vi "WS1050 16 DUT VSA-CV Sweep HD_Cycling_Ver1.0.vi"() -> ()   [LabVIEW 2012]
uses:
  Type Defs/WSVCAP SHL I2C DUT Mask Mode Enum.ctl
  <vilib>/Utility/file.llb/Read From Spreadsheet File (DBL).vi
  SubVI/Agilent E363X Series/Agilent E363X Series.lvlib
  SubVI/keithley_2000/Keithley 2000/Keithley 2000.lvlib
  SubVI/2012_Keithley 24XX/Keithley 24XX.lvlib
panel:
  out "VISA resource name out":refnum<visa-resource-name>="GPIB0::3::INSTR"
  out "date string":string="5/19/2014"
  out "PS1 Out":refnum<visa-resource-name>
  out "Ke2000 Out":refnum<visa-resource-name>="GPIB0::9::INSTR"
  in  "Tab Control":enum32{"Inst Control", "Data Output", "Graphs"}(tab)
  out "AD7747 Values":string[][](table)
  in  "Lot#":string="4NEMB"
  in  "Wafer#":string="20-EB"
  in  "File Name":string="HD_4NEMB_25_EB_65C_44V_100DC_BRD2_150916_1"
  in  "TMN DC\\CAP Data Log File Path":path=path "C:/WS1050 16 DUT Data"
  in  "SN":string[](array[string])=["1", "2", "3", "4", "5", "6", "7", "8", "9", "10", "11", "12", "13", "14", "15", "16"]
  in  "Test Program":string="WS1050 16 DUT VSA_CV Sweep HD_Cycling Ver1.0"
  out "Current Date":string="8/28/2014"
  out "Current Time":string="0950"
  in  "Start Date":string="4/24/2014"
  in  "Start Time":string="1542"
  in  "Comment":string="VSA CV Sweep"
  in  "OK Button":bool
  in  "Calibration":bool
  in  "Control Setting":bool
  in  "CP Setting":i32(ring) items=["CP OFF", "CP ON", "CP 35V", "CP 40V", "CP 44V", "CP 50V", "DVA OFF", "DVA ON", "Reg1 ON", "Reg1 OFF", "Reg2 ON", "Reg2 OFF", "Reg3 ON", "Reg3 OFF"]
  in  "VDD(V)":dbl=3.3 format="%.3g"
  in  "SPI Clock Rate (Hz)":dbl=1000000.0 caption="Meas Speed" format="%.1p Hz"
  out "AR  Measurent(Hz)":dbl
  in  "PS1 Source":refnum<visa-resource-name>="GPIB0::5::INSTR"
  in  "Ke2000":refnum<visa-resource-name>="GPIB0::9::INSTR"
  out "Simulate FPGA":bool
  out "Online":bool
  in  "Ke2400":refnum<visa-resource-name>="GPIB0::3::INSTR"
  in  "Initialize AD7747":bool
  in  "DUT Mask Mode":T1=enum."All"
  in  "RFFE Slave Address":u8=7 caption="Slave Address" format="0x%02x"
  out "Activity Log":string="05/19/2014 -- 12:24:35.853::WSVCAP::APP::Application Started\n05/19/2014 -- 12:24:37.606::WSVCAP::WSVCAP SHL::WR I2C-REG:0x0A;MASK:0xFFFFFFFFFFFF;C1 DATA:22:22:22:22:22:22:22:22:22:22:22:22:22:22:22:22;C2 DATA:22:22:22:22:22:22:22:22:22:22:22:22:22:22:22:22;C3 DATA:22:22:22:22:22:22:22:22:22:22:22:22:22:22:22:22\r\n05/19/2014 -- 12:24:37.773::WSVCAP::WSVCAP SHL::WR I2C-ST:0,0,4,1\r\n05/19/2014 -- 12:24:37.903::WSVCAP::WSVCAP SHL::RD I2C-BYTES:4;ADD:0x00;MASK:0xFFFFFFFFFFFF\r\n05/19/2014 -- 12:24:38.045::WSVCAP::WSVCAP SHL::RD I2C:C1 DATA:2:2:2:2:2:2:2:2:2:2:2:2:2:2:2:2|A7:A9:AA:82:82:7F:82:81:82:81:83:82:81:82:82:81|46:36:BB:88:44:A3:E9:2B:32:20:ED:25:BB:3D:68:B|2C:6A:EB:A7:22:56:FE:CC:36:82:D7:B0:3B:48:F9:CC;C2 DATA:2:2:2:2:2:2:2:2:2:2:2:2:2:2:2:2|94:94:94:80:80:80:80:80:81:7E:7E:81:80:7E:80:80|47:33:15:82:62:B:E8:1C:D7:C3:7D:41:7C:B7:4C:2A|C4:B4:AE:8:1E:D1:4E:37:11:C0:6F:63:42:9D:63:B5;C3 DATA:2:2:2:2:2:2:2:2:2:2:2:2:2:2:2:2|95:95:95:81:81:7E:81:80:84:7D:80:83:81:7E:7F:80|AB:C4:14:B5:7B:52:DF:C9:79:5D:5F:30:99:31:1E:F4|6E:5C:F7:A8:C3:EB:7B:EF:33:92:89:77:4D:67:75:DD;STATUS:0:0:4:0\r\n05/19/2014 -- 12:24:38.046::WSVCAP::WSVCAP SHL::WR I2C-REG:0x0A;MASK:0xFFFFFFFFFFFF;C1 DATA:22:22:22:22:22:22:22:22:22:22:22:22:22:22:22:22;C2 DATA:22:22:22:22:22:22:22:22:22:22:22:22:22:22:22:22;C3 DATA:22:22:22:22:22:22:22:22:22:22:22:22:22:22:22:22\r\n05/19/2014 -- 12:24:38.089::WSVCAP::WSVCAP SHL::WR I2C-ST:0,0,4,1\r\n05/19/2014 -- 12:24:38.219::WSVCAP::WSVCAP SHL::RD I2C-BYTES:4;ADD:0x00;MASK:0xFFFFFFFFFFFF\r\n05/19/2014 -- 12:24:38.362::WSVCAP::WSVCAP SHL::RD I2C:C1 DATA:2:2:2:2:2:2:2:2:2:2:2:2:2:2:2:2|A7:AB:AA:82:82:82:83:83:82:82:82:82:7F:82:82:81|4B:32:96:83:3E:61:43:17:25:62:AB:4D:A2:40:2E:5|3C:76:2B:B4:EE:E4:A9:1A:AA:A:26:C7:21:2E:87:5B;C2 DATA:2:2:2:2:2:2:2:2:2:2:2:2:2:2:2:2|94:94:94:80:80:80:80:80:80:7F:80:81:80:80:7F:80|4A:32:19:7D:19:6C:79:46:61:7F:4B:B8:A5:30:F3:14|B4:70:A:8C:9C:DC:43:FA:1E:A:C6:21:A:A9:13:F3;C3 DATA:2:2:2:2:2:2:2:2:2:2:2:2:2:2:2:2|95:97:94:81:80:81:82:81:80:7E:81:84:7F:81:80:80|B2:32:D0:A7:9E:4C:AB:D4:EE:D9:F0:82:B7:91:7:FF|C1:91:B6:3D:D8:E:1B:4F:9F:6A:F1:6C:E7:3F:7:BA;STATUS:0:0:4:0\r\n05/19/2014 -- 12:24:38.364::WSVCAP::WSVCAP SHL::WR I2C-REG:0x0A;MASK:0xFFFFFFFFFFFF;C1 DATA:22:22:22:22:22:22:22:22:22:22:22:22:22:22:22:22;C2 DATA:22:22:22:22:22:22:22:22:22:22:22:22:22:22:22:22;C3 DATA:22:22:22:22:22:22:22:22:22:22:22:22:22:22:22:22\r\n05/19/2014 -- 12:24:38.406::WSVCAP::WSVCAP SHL::WR I2C-ST:0,0,4,1\r\n05/19/2014 -- 12:24:38.536::WSVCAP::WSVCAP SHL::RD I2C-BYTES:4;ADD:0x00;MASK:0xFFFFFFFFFFFF\r\n05/19/2014 -- 12:24:38.678::WSVCAP::WSVCAP SHL::RD I2C:C1 DATA:2:2:2:2:2:2:2:2:2:2:2:2:2:2:2:2|A7:A9:AB:82:82:81:82:82:82:82:82:82:82:82:82:81|46:71:4C:87:43:3D:7F:FC:25:4F:8E:54:97:3E:60:8C|AA:F4:1F:B5:CE:43:1F:36:9:87:9C:78:86:5:B6:8E;C2 DATA:2:2:2:2:2:2:2:2:2:2:2:2:2:2:2:2|94:94:94:80:7F:7F:80:80:80:80:80:81:80:80:80:80|49:36:18:7D:6E:C5:E4:3C:81:2E:41:D3:75:71:E3:72|E8:D3:E6:D1:E0:48:AE:D4:54:D:E8:8E:B4:41:68:4;C3 DATA:2:2:2:2:2:2:2:2:2:2:2:2:2:2:2:2|95:95:95:81:7F:7F:81:81:81:81:81:84:81:81:82:81|B3:F5:90:AB:82:69:7B:93:D0:77:E8:D5:E8:8C:84:E8|B9:AC:EE:2B:B6:71:8F:4A:74:31:56:BB:8A:B7:A0:C8;STATUS:0:0:4:0\r\n05/19/2014 -- 12:24:38.681::WSVCAP::WSVCAP SHL::WR I2C-REG:0x0A;MASK:0xFFFFFFFFFFFF;C1 DATA:22:22:22:22:22:22:22:22:22:22:22:22:22:22:22:22;C2 DATA:22:22:22:22:22:22:22:22:22:22:22:22:22:22:22:22;C3 DATA:22:22:22:22:22:22:22:22:22:22:22:22:22:22:22:22\r\n05/19/2014 -- 12:24:38.723::WSVCAP::WSVCAP SHL::WR I2C-ST:0,0,4,1\r\n05/19/2014 -- 12:24:38.854::WSVCAP::WSVCAP SHL::RD I2C-BYTES:4;ADD:0x00;MASK:0xFFFFFFFFFFFF\r\n05/19/2014 -- 12:24:38.996::WSVCAP::WSVCAP SHL::RD I2C:C1 DATA:2:2:2:2:2:2:2:2:2:2:2:2:2:2:2:2|A7:A9:AA:82:82:7F:83:81:82:81:84:82:7F:82:7F:82|43:FB:E:7F:3C:AD:35:35:26:A2:6C:21:4B:3D:8:6|63:9A:E1:F3:95:32:91:42:90:3C:78:1F:5C:D7:5F:D8;C2 DATA:2:2:2:2:2:2:2:2:2:2:2:2:2:2:2:2|94:94:94:80:80:80:80:80:81:80:7E:81:80:7E:7F:80|48:36:18:7F:5E:3D:69:83:DE:AE:A1:9E:31:AE:BB:96|15:A0:44:17:13:FD:CC:C8:6D:B2:EF:A7:C:C7:3B:F;C3 DATA:2:2:2:2:2:2:2:2:2:2:2:2:2:2:2:2|95:96:94:81:81:7E:82:80:84:80:80:84:7F:7E:7D:82|AD:3B:6D:A9:7C:57:9D:F5:7A:96:23:5C:36:2D:ED:5A|CD:46:DB:3B:C7:BD:70:60:33:B8:B:F7:63:A:51:4D;STATUS:0:0:4:0\r\n05/19/2014 -- 12:24:38.998::WSVCAP::WSVCAP SHL::WR I2C-REG:0x0A;MASK:0xFFFFFFFFFFFF;C1 DATA:22:22:22:22:22:22:22:22:22:22:22:22:22:22:22:22;C2 DATA:22:22:22:22:22:22:22:22:22:22:22:22:22:22:22:22;C3 DATA:22:22:22:22:22:22:22:22:22:22:22:22:22:22:22:22\r\n05/19/2014 -- 12:24:39.040::WSVCAP::WSVCAP SHL::WR I2C-ST:0,0,4,1\r\n05/19/2014 -- 12:24:39.170::WSVCAP::WSVCAP SHL::RD I2C-BYTES:4;ADD:0x00;MASK:0xFFFFFFFFFFFF\r\n05/19/2014 -- 12:24:39.311::WSVCAP::WSVCAP SHL::RD I2C:C1 DATA:2:2:2:2:2:2:2:2:2:2:2:2:2:2:2:2|A7:AA:AB:82:82:81:82:81:82:81:82:82:82:82:7F:82|44:F1:90:87:45:44:C8:2C:2C:F1:FC:1B:94:3B:3C:75|4A:49:95:19:99:73:64:3:23:24:F3:A2:5E:7F:C4:B6;C2 DATA:2:2:2:2:2:2:2:2:2:2:2:2:2:2:2:2|94:94:94:80:80:80:80:7F:80:80:7E:80:80:7E:7F:80|4C:36:17:7D:A8:9F:DE:C7:53:6D:8A:F4:41:A5:C6:E0|90:2E:24:C:D9:22:E4:76:3B:40:1D:53:33:B1:3E:4D;C3 DATA:2:2:2:2:2:2:2:2:2:2:2:2:2:2:2:2|95:97:95:81:81:7F:81:80:80:81:7F:82:81:7E:7D:82|AE:2B:A7:AB:CC:CD:A4:38:FD:17:80:F2:92:2D:45:C4|76:E5:D:B9:AD:B5:BA:8D:28:32:9E:42:B7:20:4A:D9;STATUS:0:0:4:0\r\n05/19/2014 -- 12:24:39.313::WSVCAP::WSVCAP SHL::WR I2C-REG:0x0A;MASK:0xFFFFFFFFFFFF;C1 DATA:22:22:22:22:22:22:22:22:22:22:22:22:22:22:22:22;C2 DATA:22:22:22:22:22:22:22:22:22:22:22:22:22:22:22:22;C3 DATA:22:22:22:22:22:22:22:22:22:22:22:22:22:22:22:22\r\n05/19/2014 -- 12:24:39.355::WSVCAP::WSVCAP SHL::WR I2C-ST:0,0,4,1\r\n05/19/2014 -- 12:24:39.486::WSVCAP::WSVCAP SHL::RD I2C-BYTES:4;ADD:0x00;MASK:0xFFFFFFFFFFFF\r\n05/19/2014 -- 12:24:39.628::WSVCAP::WSVCAP SHL::RD I2C:C1 DATA:2:2:2:2:2:2:2:2:2:2:2:2:2:2:2:2|A7:A9:AA:82:82:82:83:82:82:82:82:82:7F:82:7F:82|47:18:E4:87:3E:E7:6:65:25:92:37:38:A8:3E:89:85|7C:A7:7:2B:A3:7A:EC:EF:89:ED:F4:D3:D8:BC:3A:F5;C2 DATA:2:2:2:2:2:2:2:2:2:2:2:2:2:2:2:2|94:94:94:80:7F:80:80:7F:81:80:7E:80:80:80:81:80|49:37:17:80:76:25:6A:F8:DF:55:97:4D:B8:5B:2B:B1|13:E3:9A:3E:1A:2D:4F:B6:DB:E9:61:FA:8B:D6:9:CC;C3 DATA:2:2:2:2:2:2:2:2:2:2:2:2:2:2:2:2|95:95:95:81:7F:80:82:81:84:80:7F:81:80:81:7F:82|AF:93:3B:AF:5B:11:82:E4:7E:C3:2D:72:9:96:D9:A|DB:96:F2:10:5F:64:9A:C6:98:12:27:7D:10:D3:20:D9;STATUS:0:0:4:0\r\n05/19/2014 -- 12:24:40.132::WSVCAP::WSVCAP SHL::CLOSE\r\n"
  in  "C1 Cap DAC":u8=128 caption="B Data In" format="0x%02x"
  in  "C2 Cap DAC":u8=128 caption="B Data In" format="0x%02x"
  in  "C3 Cap DAC":u8=128 caption="B Data In" format="0x%02x"
  out "IDD Brd(uA)":string
  in  "VSA_IDD(A)":dbl=0.1
  in  "Cmd to HD_ON":string="0702013B3B3B"
  in  "Stress Voltage(V)":dbl=10.0
  in  "error in (no error)":errorcluster
  out "error out":errorcluster
  in  "CP to HD/Cycle":i32(ring)=4 items=["CP HDC 35V", "CP HDC 40.25V", "CP HDC 27.5V", "CP HDC 30.5V", "CP HDC 44V", "CP HDC 50V"]
  out "STATUS":string="Idle...."
  in  "stop":bool
  out "VSA_C1_T0":string[](array[string])
  out "VSA_Value(pF)":string[][](array[string])
  out "VSA_C3_T0":string[](array[string])
  out "VSA_C2_T0":string[](array[string])
  in  "Abort":bool
  out "error out 2":errorcluster
  in  "Set HD Time \nto Complete(Min)":u64=259200
  out "HD Time\nCompleted(Min)":u64
  out "Verify Test Condition":string[](array[string])
  out "All CMin Current":string[][](table)
  out "Previous Time":string="12:20:26 PM"
  out "Running Loops":i32=1
  out "Verify Drivers to Stress":string[](array[string])
  out "VSA Delta C1(pF)":dbl[](array[numeric])
  out "VSA Delta C2(pF)":dbl[](array[numeric])
  out "VSA Delta C3(pF)":dbl[](array[numeric])
  out "CP Current(uA)":string[](array[string])
  out "Plot VSA Delta C3":cluster{dbl[], "VSA Delta C(pF)":dbl[]}(graph)
  out "Plot VSA Delta C2":cluster{dbl[], "VSA Delta C(pF)":dbl[]}(graph)
  out "Plot VSA Delta C1":cluster{dbl[], "VSA Delta C(pF)":dbl[]}(graph)
  # "Company:  WiSpry Inc 20 Fairbanks \nSte 198 Irvine CA 92618\n\nAuthor:  Andy V Tran\nCreated:  09/18/2015\nLabVIEW 2012 Pro\nTP:  WS1050 16 DUT VSA_CV Sweep HD_Cycling Ver1.0\nFPGA Version: WS_VCAP Driver 024"
  # "Note:  Ver1.0 is a original version.\n\n1.  Two look up tables, \n      a.  1st is for Stress\n      b.  2nd is for Voltage sweep"
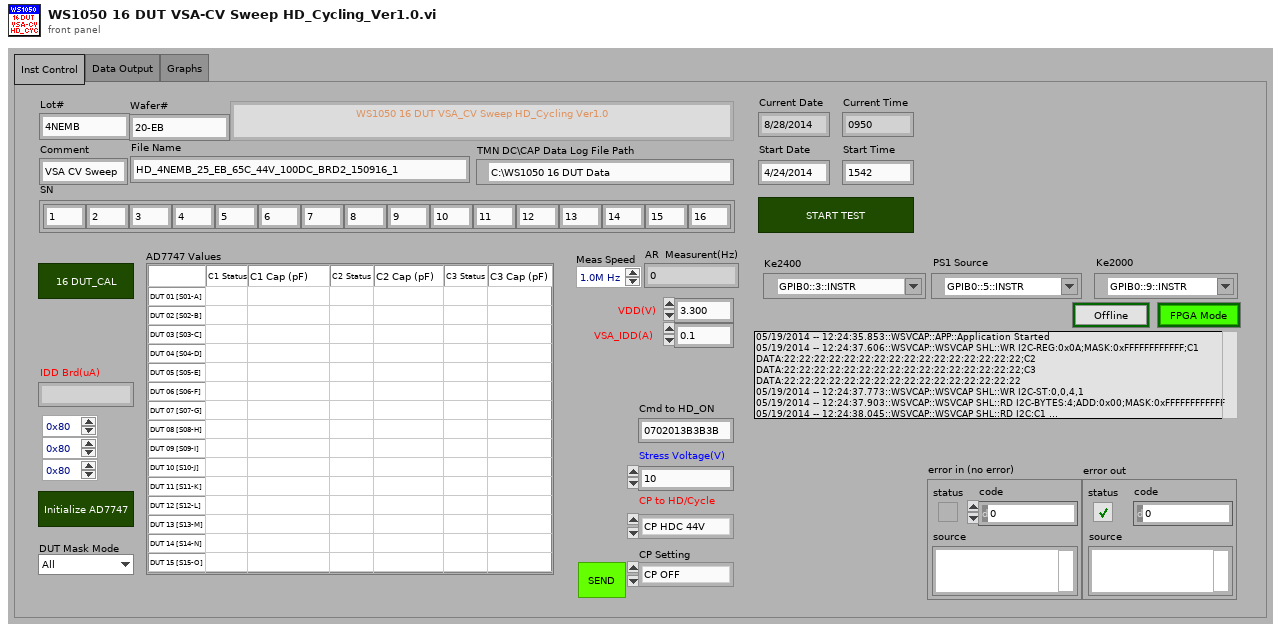
[diagram p1: front panel]
types:
  T1 = typedef "WSVCAP SHL I2C DUT Mask Mode Enum.ctl" = enum16{"Custom", "C1", "C2", "C3", "All"}
  T2 = typedef "WSVCAP SHL Core System Cluster.ctl" = cluster{"Settings":T3, "FPGA Resource":tag, "Online":bool, "I2C Wait Ticks":u32, "SPI Wait Ticks":u32, "RFFE Wait Ticks":u32}
  T3 = typedef "WSVCAP SHL I2C Settings Cluster.ctl" = cluster{"FPGA Resource Name":string, "I2C Slave Address":u8, "I2C Clock Rate (Hz)":dbl, "SPI Clock Rate (Hz)":dbl, "RFFE Slave Address":u8, "RFFE Clock Rate (Hz)":dbl, "Simulate FPGA":bool, "C1 Cap DAC Default":u8, "C2 Cap DAC Default":u8, "C3 Cap DAC Default":u8}
  T4 = enum16{"Idle...", "Voltage 1", "Voltage 2", "Voltage 3"}[]
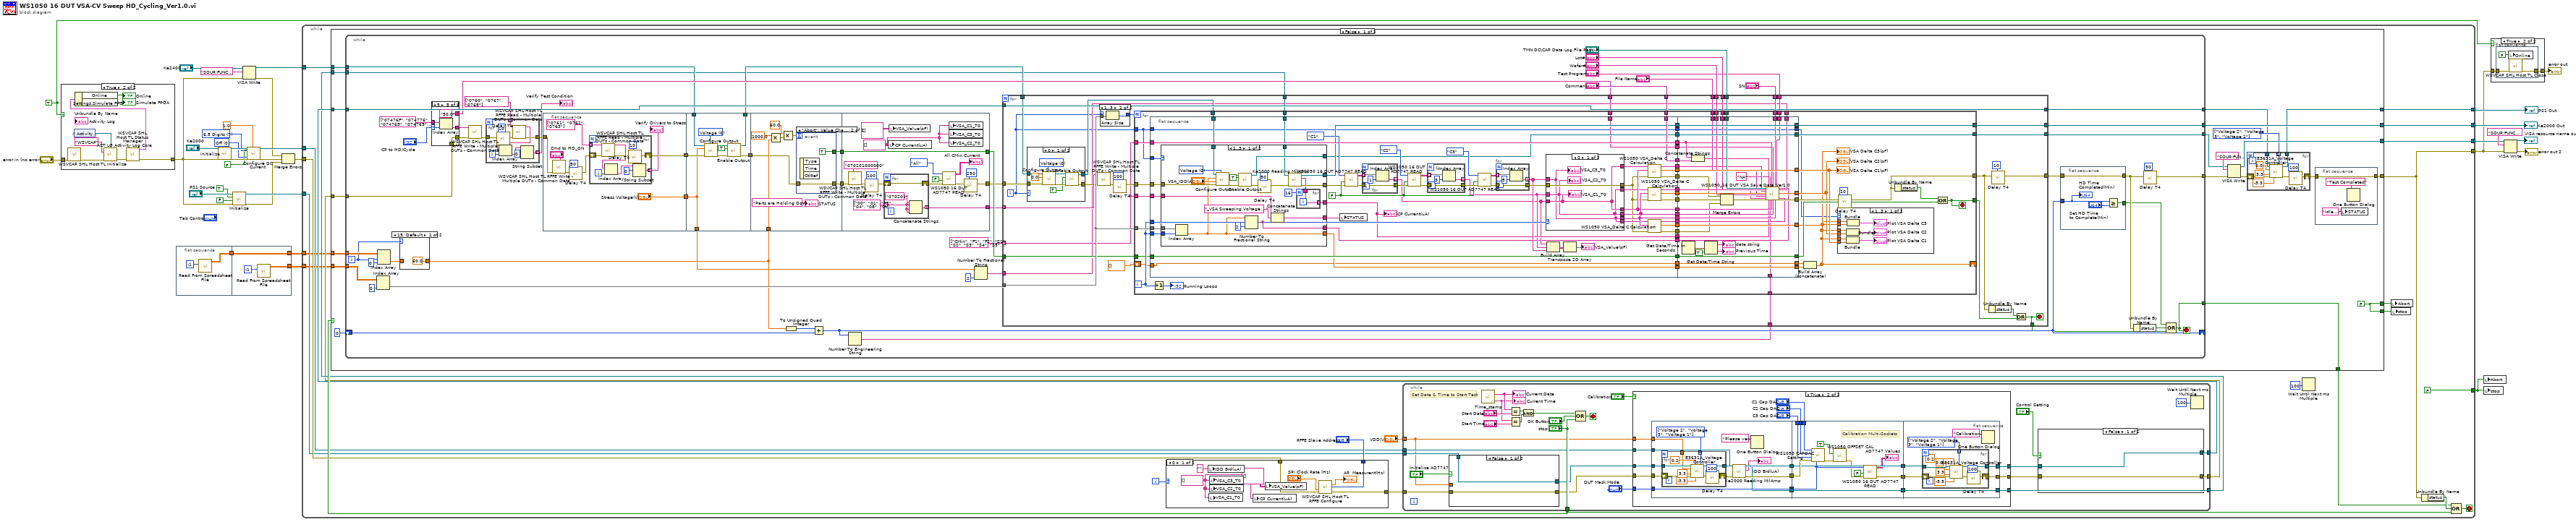
[diagram p0: block diagram]
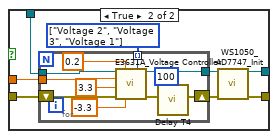
[diagram p5: hidden frame]
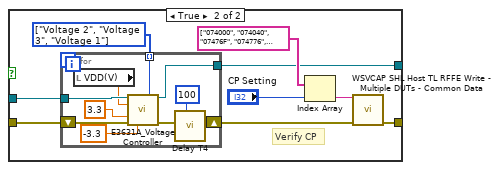
[diagram p6: hidden frame]
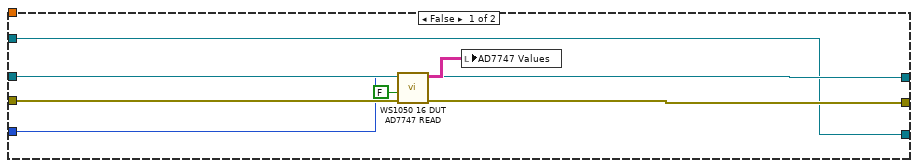
[diagram p7: hidden frame]
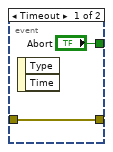
[diagram p9: hidden frame]
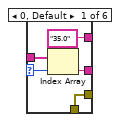
[diagram p10: hidden frame]
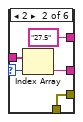
[diagram p11: hidden frame]
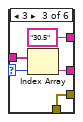
[diagram p12: hidden frame]
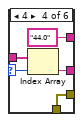
[diagram p13: hidden frame]
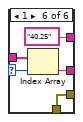
[diagram p14: hidden frame]
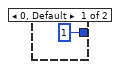
[diagram p15: hidden frame]
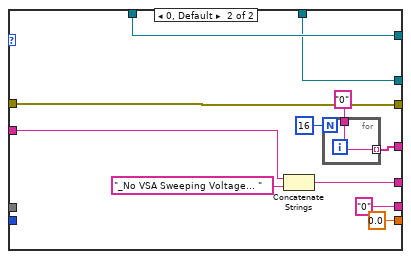
[diagram p18: hidden frame]
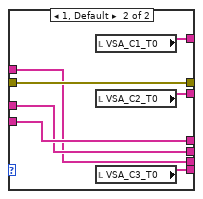
[diagram p19: hidden frame]
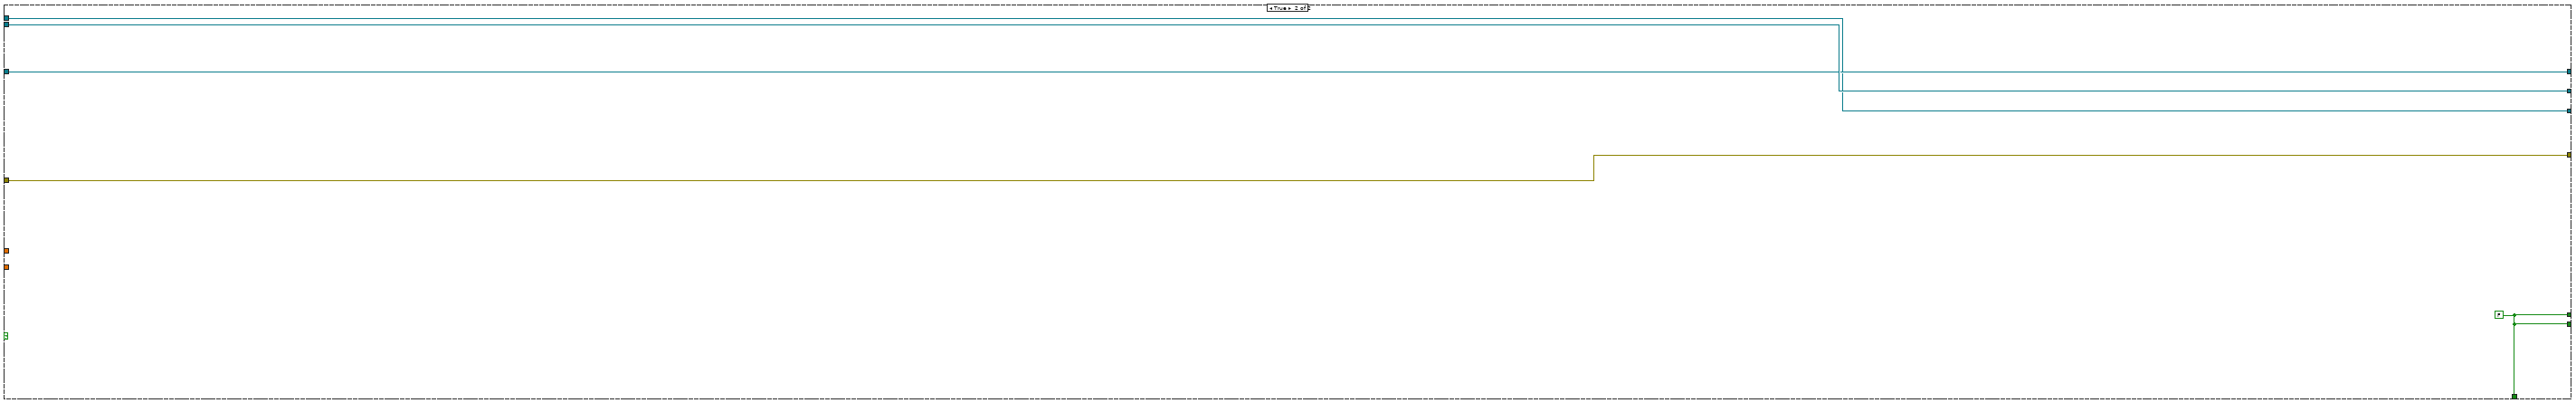
[diagram p20: hidden frame]
diagram:
  w20 = TRUE
  w26 = u16 0 items=["Off", "Moving Filter", "Repeating Filter"] ("Digital Filter (0: Off)")
  w27 = u16 7 items=["3.5 Digits"=4, "4.5 Digits"=5, "5.5 Digits"=6, "6.5 Digits"=7] ("Resolution (7: 6.5 digits)")
  n1 = case shown="True" w20 {
    tunnel: "error in (no error)" -> [w35 w36]
    tunnel: [w35 w43] -> w9
    frame False {
    }
    frame True {
      n2 = call "WSVCAP SHL Host TL Initialize.vi"("error in"=w36) -> ("error out"=w37:errorcluster)  [unwired: 13 in, 1 out]
      n3 = control-ref of="Activity Log"() -> (w39:refnum<vi>)
      n4 = call "ACT LG Activity Log Core.vi"("Display Ref"=w39, "Source"="WSVCAP", "Error In (no error)"=w37) -> ("Error Out"=w38:errorcluster)  [unwired: 11 in, 1 out]
      n5 = call "WSVCAP SHL Host TL Status Manager.vi"("error in"=w38) -> ("System Out"=w44:T2, "error out"=w43:errorcluster)  [unwired: 13 in]
      n6 = Unbundle By Name(w44) -> ("Online"=→"Online":bool, "Settings.Simulate FPGA"=→"Simulate FPGA":bool)
    }
  }
  n7 = flat-sequence {
    tunnel: [w46] -> w4
    tunnel: w4 -> [w49]
    tunnel: [w49] -> w3
    tunnel: [w48] -> w2
    frame #0 {
      n8 = call-poly <vilib>:"Read From Spreadsheet File.vi"("number of rows (all:-1)"=-1) -> ("all rows"=w46:dbl[][])  [unwired: 6 in, 4 out]
    }
    frame #1 {
      n9 = call-poly <vilib>:"Read From Spreadsheet File.vi"("number of rows (all:-1)"=-1) -> ("all rows"=w48:dbl[][])  [unwired: 6 in, 4 out]
    }
  }
  n10 = call "Initialize.vi"("VISA resource name"="Ke2000", "error in (no error)"=w9) -> ("VISA resource name out"=w29:refnum<visa-resource-name>, "error out"=w28:errorcluster)  [unwired: 16 in]
  n11 = call "Initialize.vi"("error in (no error)"=w9, "Reset? (T: Yes)"=FALSE, "ID Query? (T: Yes)"=TRUE, "VISA resource name"="PS1 Source") -> ("error out"=w8:errorcluster, "VISA resource name out"=w32:refnum<visa-resource-name>)  [unwired: 6 in]
  n12 = VISA Write(VISA resource name="Ke2400", write buffer="SOUR:FUNC VOLT;VOLT:MODE FIX;RANG 100;LEV 0.0;:SENS:FUNC \"CURR\";CURR:PROT 60E-3;RANG 100E-3;:OUTP ON", error in (no error)=w9) -> (VISA resource name out=w17:refnum<visa-resource-name>, error out=w12:errorcluster)  [unwired: 1 out]
  n13 = call "Configure DC Current.vi"("VISA resource name"=w29, "Resolution (7: 6.5 digits)"=w27, "error in (no error)"=w28, "Auto Range? (T: Auto)"=FALSE, "Digital Filter (0: Off)"=w26, "Custom Range (0 A)"=1.0) -> ("VISA resource name out"=w24:refnum<visa-resource-name>, "error out"=w10:errorcluster)  [unwired: 12 in]
  n14 = Merge Errors(w12, w10, w8) -> (w18:errorcluster)
  n15 = while {
    tunnel: w18 -> [w68]
    tunnel: [w57] -> w14
    tunnel: w32 -> [w61]
    tunnel: w24 -> [w62]
    tunnel: [w71] -> w23
    tunnel: [w70] -> w22
    tunnel: w17 -> [w67]
    tunnel: [w66] -> w15
    tunnel: [FALSE] -> w7
    tunnel: w3 -> [w53]
    tunnel: w2 -> [w52]
    i -> [w69]
    stop <- w72 stop-if-true
    n16 = case shown="0" w69 {
      tunnel: w68 -> [w82 w83]
      tunnel: [w81 w83] -> w64
      tunnel: "RFFE Slave Address" -> [w79 _]
      frame 0 {
        w76 = string[] []
        n17 = local write "IDD Brd(uA)"("" ("uA")) -> ()
        n18 = local write "VSA_C1_T0"(w76) -> ()
        n19 = local write "VSA_C3_T0"(w76) -> ()
        n20 = local write "VSA_C2_T0"(w76) -> ()
        n21 = local write "CP Current(uA)"(w76) -> ()
        n22 = local write "VSA_Value(pF)"(string[][] []) -> ()
        n23 = call "WSVCAP SHL Host TL RFFE Configure.vi"("RFFE Slave Address"=w79, "Clock Rate (Hz)"="SPI Clock Rate (Hz)", "error in"=w82) -> ("Actual Rate (Hz)"=→"AR  Measurent(Hz)":dbl, "error out"=w81:errorcluster)  [unwired: 11 in]
      }
      frame 1, Default {
      }
    }
    n24 = while {
      tunnel: ["stop"] -> w65
      tunnel: w64 -> [w95]
      tunnel: [w87] -> w58
      tunnel: w61 -> [w93]
      tunnel: w62 -> [w89]
      tunnel: [w90] -> w60
      tunnel: [w88] -> w59
      tunnel: "VDD(V)" -> [w85]
      stop <- w102 stop-if-true
      # "Set Date & Time to Start Test"
      n25 = case shown="False" "Initialize AD7747" {
        tunnel: w95 -> [w111 w117]
        tunnel: [w111 w113] -> w94
        tunnel: w93 -> [w110 w115]
        tunnel: [w110 w114] -> w92
        tunnel: w85 -> [_ w112]
        frame False {
        }
        frame True {
          w118 = T4 [enum."Voltage 2", enum."Voltage 3", enum."Voltage 1"] items=["Idle...", "Voltage 1", "Voltage 2", "Voltage 3"]
          n26 = for {
            tunnel: w115 -> [w128]
            tunnel: w118 -> [w126] mode=indexing
            tunnel: [w125] -> w114
            shift-right: [w122] -> w116
            shift-left: w117 -> [w129]
            tunnel: w112 -> [w120]
            n27 = call "E3631A_Voltage Controller.vi"("VISA resource name"=w128, "I_VDD(A)"=0.2, "Channel Controller"=w126, "Voltage 1"=w120, "Voltage 2"=3.3, "error in (no error)"=w129, "Voltage 3"=-3.3) -> ("VISA resource name out"=w125:refnum<visa-resource-name>, "error out"=w121:errorcluster)  [unwired: 7 in]
            n28 = call "Delay T4.vi"("milliseconds to wait"=u32 100, "error in (no error)"=w121) -> ("error out"=w122:errorcluster)  [unwired: 9 in]
          }
          n29 = call "WS1050_AD7747_Init.vi"("error in"=w116) -> ("error out"=w113:errorcluster)  [unwired: 10 in]
        }
      }
      n30 = call "Time_stamp.vi"() -> ("date/time string"=w107:string, "date string"=w109:string)  [unwired: 2 in]
      "Current Date" <- w109
      "Current Time" <- w107
      n31 = Equal?(x=w109, y="Start Date") -> (x = y?=w105:bool)
      n32 = Equal?(x=w107, y="Start Time") -> (x = y?=w104:bool)
      n33 = And(x=w105, y=w104) -> (x .and. y?=w101:bool)
      n34 = Compound Arithmetic op=OR(w101, "OK Button", "stop") -> (w102:bool)
      n35 = case shown="True" "Calibration" {
        tunnel: w94 -> [w156 w175]
        tunnel: [w155 w172] -> w86
        tunnel: w92 -> [w154 w171]
        tunnel: "DUT Mask Mode" -> [w153 w167]
        tunnel: [w154 w166] -> w91
        tunnel: w89 -> [w152 w162]
        tunnel: [w152 w159] -> w88
        tunnel: w85 -> [_ w158]
        frame False {
          n36 = call "WS1050 16 DUT AD7747 READ.vi"("error in"=w156, "Log (T)"=FALSE, "DUT Mask Mode (All)"=w153) -> ("error out"=w155:errorcluster, "AD7747 Values"=w157:string[][])  [unwired: 7 in]
          n37 = local write "AD7747 Values"(w157) -> ()
        }
        frame True {
          n38 = flat-sequence {
            tunnel: w175 -> [w185]
            tunnel: [w180] -> w174
            tunnel: w171 -> [w184]
            tunnel: [w183] -> w170
            tunnel: w167 -> [w182]
            tunnel: [w182] -> w168
            tunnel: w162 -> [w178]
            tunnel: [w177] -> w161
            tunnel: w158 -> [w176]
            tunnel: w174 -> [w211]
            tunnel: [w210] -> w173
            tunnel: w170 -> [w209]
            tunnel: [w209] -> w169
            tunnel: w168 -> [w208]
            tunnel: "C1 Cap DAC" -> [w204]
            tunnel: "C2 Cap DAC" -> [w203]
            tunnel: "C3 Cap DAC" -> [w202]
            tunnel: w161 -> [w201]
            tunnel: [w201] -> w160
            tunnel: w173 -> [w214]
            tunnel: [w217] -> w172
            tunnel: w169 -> [w216]
            tunnel: [w213] -> w166
            tunnel: w160 -> [w212]
            tunnel: [w212] -> w159
            frame #0 {
              w186 = T4 [enum."Voltage 2", enum."Voltage 3", enum."Voltage 1"] items=["Idle...", "Voltage 1", "Voltage 2", "Voltage 3"]
              n39 = for {
                tunnel: w184 -> [w197]
                tunnel: w186 -> [w194] mode=indexing
                tunnel: [w193] -> w183
                shift-right: [w191] -> w179
                shift-left: w185 -> [w198]
                tunnel: w176 -> [w188]
                n40 = call "E3631A_Voltage Controller.vi"("VISA resource name"=w197, "I_VDD(A)"=0.2, "Channel Controller"=w194, "Voltage 1"=w188, "Voltage 2"=3.3, "error in (no error)"=w198, "Voltage 3"=-3.3) -> ("VISA resource name out"=w193:refnum<visa-resource-name>, "error out"=w190:errorcluster)  [unwired: 7 in]
                n41 = call "Delay T4.vi"("milliseconds to wait"=u32 100, "error in (no error)"=w190) -> ("error out"=w191:errorcluster)  [unwired: 9 in]
              }
              n42 = call "Ke2000 Reading MilAmp.vi"("error in (no error)"=w179, "VISA resource name"=w178) -> ("error out"=w180:errorcluster, "uA"=→"IDD Brd(uA)":string, "VISA resource name out"=w177:refnum<visa-resource-name>)  [unwired: 7 in]
              n43 = One Button Dialog(message="Please verify all sockets should be empty...") -> ()  [unwired: 1 in, 1 out]
            }
            frame #1 {
              # "Calibration Multi-Sockets"
              n44 = call "WS1050 CAPDAC Setting.vi"("DUT Mask Mode (All)"=w208, "error in"=w211, "C3 Cap DAC"=w202, "C2 Cap DAC"=w203, "C1 Cap DAC"=w204) -> ("error out"=w206:errorcluster)  [unwired: 5 in, 1 out]
              n45 = call "WS1050 OFFSET CAL.vi"("error in"=w206, "OFFSET CAL"=TRUE ("Read?")) -> ("error out"=w205:errorcluster)  [unwired: 8 in, 1 out]
              n46 = call "WS1050 16 DUT AD7747 READ.vi"("error in"=w205, "Log (T)"=FALSE, "DUT Mask Mode (All)"=w208) -> ("error out"=w210:errorcluster, "AD7747 Values"=→"AD7747 Values":string[][])  [unwired: 7 in]
            }
            frame #2 {
              w215 = T4 [enum."Voltage 2", enum."Voltage 3", enum."Voltage 1"] items=["Idle...", "Voltage 1", "Voltage 2", "Voltage 3"]
              n47 = for {
                tunnel: w216 -> [w229]
                tunnel: w215 -> [w225] mode=indexing
                tunnel: [w224] -> w213
                shift-right: [w220] -> w217
                shift-left: w214 -> [w226]
                n48 = call "E3631A_Voltage Controller.vi"("VISA resource name"=w229, "I_VDD(A)"=0.2, "Channel Controller"=w225, "Voltage 1"=0.0, "Voltage 2"=3.3, "error in (no error)"=w226, "Voltage 3"=-3.3) -> ("VISA resource name out"=w224:refnum<visa-resource-name>, "error out"=w219:errorcluster)  [unwired: 7 in]
                n49 = call "Delay T4.vi"("milliseconds to wait"=u32 100, "error in (no error)"=w219) -> ("error out"=w220:errorcluster)  [unwired: 9 in]
              }
              n50 = One Button Dialog(message="Calibration Completed....") -> ()  [unwired: 1 in, 1 out]
            }
          }
        }
      }
      n51 = case shown="False" "Control Setting" {
        tunnel: [w130 w133] -> w87
        tunnel: w91 -> [w131 w136]
        tunnel: [w131 w134] -> w90
        tunnel: w86 -> [w130 w132]
        frame False {
        }
        frame True {
          w137 = T4 [enum."Voltage 2", enum."Voltage 3", enum."Voltage 1"] items=["Idle...", "Voltage 1", "Voltage 2", "Voltage 3"]
          # "Verify CP"
          n52 = for {
            tunnel: w136 -> [w149]
            tunnel: w137 -> [w146] mode=indexing
            shift-right: [w143] -> w135
            shift-left: w132 -> [w150]
            tunnel: [w141] -> w134
            n53 = local read "VDD(V)"() -> (w145:dbl)
            n54 = call "E3631A_Voltage Controller.vi"("VISA resource name"=w149, "Channel Controller"=w146, "Voltage 1"=w145, "Voltage 2"=3.3, "error in (no error)"=w150, "Voltage 3"=-3.3) -> ("VISA resource name out"=w141:refnum<visa-resource-name>, "error out"=w144:errorcluster)  [unwired: 8 in]
            n55 = call "Delay T4.vi"("milliseconds to wait"=u32 100, "error in (no error)"=w144) -> ("error out"=w143:errorcluster)  [unwired: 9 in]
          }
          n56 = Index Array(array=string[] ["074000", "074040", "07476F", "074776", "07477B", "07477C", "074820", "074800", "07413B", "074100", "07423B", "074200", "07433B", "074300"], index="CP Setting") -> (element=w138:string)
          n57 = call "WSVCAP SHL Host TL RFFE Write - Multiple DUTs - Common Data.vi"("Data Out"=w138, "error in"=w135) -> ("error out"=w133:errorcluster)  [unwired: 13 in]
        }
      }
      n58 = Wait Until Next ms Multiple(millisecond multiple=u32 100) -> ()  [unwired: 1 out]
    }
    n59 = case shown="False" w65 {
      tunnel: w58 -> [w246 w702]
      tunnel: [w230 w702] -> w57
      tunnel: w60 -> [w244 w700]
      tunnel: w59 -> [w247 w701]
      tunnel: [w243 w701] -> w71
      tunnel: [w234 w700] -> w70
      tunnel: w67 -> [w249 w699]
      tunnel: [w245 w699] -> w66
      tunnel: [w242 w698] -> w55
      tunnel: [w242 w698] -> w54
      tunnel: w53 -> [w240 _]
      tunnel: w52 -> [w238 _]
      tunnel: [w233 w698] -> w50
      frame False {
        w237 = T4 [enum."Voltage 2", enum."Voltage 3", enum."Voltage 1"] items=["Idle...", "Voltage 1", "Voltage 2", "Voltage 3"]
        w242 = FALSE
        n60 = while {
          tunnel: w249 -> [w271]
          tunnel: w247 -> [w267]
          tunnel: w246 -> [w261]
          tunnel: w244 -> [w310]
          tunnel: [w309] -> w243
          tunnel: [w308] -> w235
          tunnel: [w307] -> w241
          tunnel: [w306] -> w232
          tunnel: w240 -> [w297]
          shift-right: [w288] -> _
          shift-left: u64 0 ("disabled index (col)") -> [w294]
          tunnel: w238 -> [w286]
          tunnel: [w260] -> w233
          i -> [w262]
          stop <- w260 stop-if-true
          n61 = Index Array(array=w286, index (col)=0 ("disabled index (col)")) -> (element=w285:dbl[])  [unwired: 1 in]
          n62 = Index Array(array=w297, index (row)=w262, index (col)=0 ("disabled index (col)")) -> (element=w275:dbl)
          n63 = case shown="15, Default" w262 {
            tunnel: w275 -> [_ w317]
            tunnel: [60.0 w317] -> w274
            frame 15, Default {
            }
            frame 0..14 {
            }
          }
          n64 = case shown="5" "CP to HD/Cycle" {
            selector: "CP to HD/Cycle" -> [w397 w402 w407 w412 w417 w421]
            tunnel: string[] ["07476F", "074776", "074765", "074769", "07477B", "07477C"] -> [w398 w403 w408 w413 w418 w423]
            tunnel: [w396 w401 w406 w411 w416 w422] -> w302
            tunnel: ["35.0" ("Data Out") "27.5" ("Data Out") "30.5" ("Data Out") "44.0" ("Data Out") "50.0" ("Data Out") "40.25" ("Data Out")] -> w281
            tunnel: [w394 w399 w404 w409 w414 w419] -> w301
            tunnel: w261 -> [w394 w399 w404 w409 w414 w419]
            frame 0, Default {
              n65 = Index Array(array=w398, index=w397) -> (element=w396:string)
            }
            frame 2 {
              n66 = Index Array(array=w403, index=w402) -> (element=w401:string)
            }
            frame 3 {
              n67 = Index Array(array=w408, index=w407) -> (element=w406:string)
            }
            frame 4 {
              n68 = Index Array(array=w413, index=w412) -> (element=w411:string)
            }
            frame 5 {
              n69 = Index Array(array=w418, index=w417) -> (element=w416:string)
            }
            frame 1 {
              n70 = Index Array(array=w423, index=w421) -> (element=w422:string)
            }
          }
          n71 = call "WSVCAP SHL Host TL RFFE Write - Multiple DUTs - Common Data.vi"("Data Out"=w302, "error in"=w301) -> ("error out"=w299:errorcluster)  [unwired: 13 in]
          n72 = for {
            tunnel: string[] ["0760", "0767", "0768"] -> [w391] mode=indexing
            tunnel: [w387] -> w298 mode=indexing
            tunnel: w299 -> [w385]
            tunnel: [w384] -> w292
            i -> [w390]
            n73 = call "Delay T4.vi"("milliseconds to wait"=u32 10, "error in (no error)"=w385) -> ("error out"=w392:errorcluster)  [unwired: 9 in]
            n74 = call "WSVCAP SHL Host TL RFFE Read - Multiple DUTs - Common Data.vi"("Data Out"=w391, "error in"=w392) -> ("RFFE Data In"=w389:string[], "error out"=w384:errorcluster)  [unwired: 12 in]
            n75 = Index Array(array=w389, index=w390) -> (element=w386:string)
            n76 = String Subset(string=w386, offset (0)=0) -> (substring=w387:string)  [unwired: 1 in]
          }
          "Verify Test Condition" <- w298
          n77 = flat-sequence {
            tunnel: [w323] -> w273
            tunnel: w292 -> [w329]
            tunnel: ["Stress Voltage(V)"] -> w270
            tunnel: w273 -> [w345]
            tunnel: [w346] -> w272
            tunnel: w271 -> [w344]
            tunnel: [w343] -> w269
            tunnel: w270 -> [w341]
            tunnel: [w341] -> w265
            tunnel: w272 -> [w352]
            tunnel: w274 -> [w354]
            tunnel: [w353] -> w280
            tunnel: [w351] -> w279
            tunnel: [w366] -> w278
            tunnel: [w379] -> w284
            tunnel: w280 -> [w379]
            tunnel: w279 -> [w375]
            tunnel: [w377] -> w268
            frame #0 {
              n78 = call "WSVCAP SHL Host TL RFFE Write - Multiple DUTs - Common Data.vi"("Data Out"="Cmd to HD_ON", "error in"=w329) -> ("error out"=w328:errorcluster)  [unwired: 13 in]
              n79 = call "Delay T4.vi"("milliseconds to wait"=u32 50, "error in (no error)"=w328) -> ("error out"=w325:errorcluster)  [unwired: 9 in]
              n80 = for {
                tunnel: string[] ["0761", "0762", "0763"] -> [w340] mode=indexing
                tunnel: [w336] -> w324 mode=indexing
                shift-right: [w333] -> w323
                shift-left: w325 -> [w339]
                i -> [w338]
                n81 = call "WSVCAP SHL Host TL RFFE Read - Multiple DUTs - Common Data.vi"("Data Out"=w340, "error in"=w339) -> ("RFFE Data In"=w335:string[], "error out"=w332:errorcluster)  [unwired: 12 in]
                n82 = Index Array(array=w335, index=w338) -> (element=w334:string)
                n83 = call "Delay T4.vi"("milliseconds to wait"=u32 10, "error in (no error)"=w332) -> ("error out"=w333:errorcluster)  [unwired: 9 in]
                n84 = String Subset(string=w334, offset (0)=0) -> (substring=w336:string)  [unwired: 1 in]
              }
              "Verify Drivers to Stress" <- w324
            }
            frame #1 {
              w342 = u16 0 items=["Voltage", "Current"] ("Source Mode  (0: Voltage)")
              n85 = call "Configure Output.vi"("Source Mode  (0: Voltage)"=w342, "error in (no error)"=w345, "Output Level (0)"=w341, "VISA resource name"=w344) -> ("error out"=w349:errorcluster, "VISA resource name out"=w347:refnum<visa-resource-name>)  [unwired: 6 in]
              n86 = call "Enable Output.vi"("error in (no error)"=w349, "Enable Output (T: Enable)"=TRUE, "VISA resource name"=w347) -> ("error out"=w346:errorcluster, "VISA resource name out"=w343:refnum<visa-resource-name>)  [unwired: 7 in]
            }
            frame #2 {
              n87 = Multiply(x=1000.0, y=w354) -> (x*y=w357:dbl)
              n88 = Multiply(x=60.0, y=w357) -> (x*y=w358:dbl)
              n89 = event shown="[1] \"Abort\": Value Change" {
                selector: _ -> [_ _]
                dyn-events: _ -> [_ _]
                timeout: w358 -> [_ _]
                tunnel: ["Abort" TRUE ("Abort")] -> w353
                tunnel: w352 -> [w359 w361]
                tunnel: [w359 w361] -> w351
                event Timeout {
                  n90 = event-data() -> ()  [unwired: 1 in, 2 out]
                }
                event "Abort": Value Change {
                  n91 = event-data() -> ()  [unwired: 1 in, 3 out]
                }
              }
              "STATUS" <- "Parts are Holding Down...." ("STATUS")
            }
            frame #3 {
              w373 = string[] [] ("CP Current(uA)")
              n92 = call "WSVCAP SHL Host TL RFFE Write - Multiple DUTs - Common Data.vi"("Data Out"="070201000000", "error in"=w375) -> ("error out"=w369:errorcluster)  [unwired: 13 in]
              n93 = call "Delay T4.vi"("milliseconds to wait"=u32 100, "error in (no error)"=w369) -> ("error out"=w370:errorcluster)  [unwired: 9 in]
              n94 = for {
                tunnel: string[] ["00", "01", "02", "04", "08", "0C", "10", "14", "18", "1C", "20", "24", "28", "2C", "30", "34", "38", "3B", "00"] -> [w382] mode=indexing
                tunnel: [w381] -> w377 mode=indexing
                shift-right: [w380] -> w374
                shift-left: w370 -> [w380]
                n95 = Concatenate Strings("070201" ("string"), w382, w382, w382) -> (w381:string)
              }
              n96 = local write "CP Current(uA)"(w373) -> ()
              n97 = local write "VSA_Value(pF)"(string[][] [] ("VSA_Value(pF)")) -> ()
              n98 = call "WS1050 16 DUT AD7747 READ.vi"("error in"=w374, "Log (T)"=FALSE, "DUT Mask Mode (All)"=WSVCAP_SHL_I2C_DUT_Mask_Mode_Enum."All") -> ("error out"=w365:errorcluster, "AD7747 Values"=→"All CMin Current":string[][])  [unwired: 7 in]
              n99 = local write "VSA_C1_T0"(w373) -> ()
              n100 = local write "VSA_C3_T0"(w373) -> ()
              n101 = local write "VSA_C2_T0"(w373) -> ()
              n102 = call "Delay T4.vi"("milliseconds to wait"=u32 250, "error in (no error)"=w365) -> ("error out"=w366:errorcluster)  [unwired: 9 in]
            }
          }
          n103 = To Unsigned Quad Integer(1:w274) -> (0:w295:u64)
          n104 = Add(x=w295, y=w294) -> (x+y=w288:u64)
          n105 = Number To Engineering String(4:w288) -> (0:w282:string)  [unwired: 3 in]
          n106 = Number To Fractional String(number=w265, precision (6)=i16 2) -> (F-format string=w264:string)  [unwired: 2 in]
          n107 = for {
            tunnel: w278 -> [w433]
            tunnel: [w457] -> w307
            tunnel: [w440] -> w291
            tunnel: "Comment" -> [w455]
            tunnel: "Lot#" -> [w454]
            tunnel: "Wafer#" -> [w453]
            tunnel: "SN" -> [w452]
            tunnel: "File Name" -> [w451]
            tunnel: [w450] -> w308
            tunnel: w310 -> [w450]
            tunnel: [w449] -> w309
            tunnel: w285 -> [w446]
            tunnel: w284 -> [w445]
            tunnel: [w442] -> w283
            tunnel: w282 -> [w424]
            tunnel: w281 -> [w441]
            tunnel: "TMN DC\\CAP Data Log File Path" -> [w438]
            tunnel: "Test Program" -> [w437]
            tunnel: w269 -> [w431]
            tunnel: w268 -> [w435] mode=indexing
            tunnel: w267 -> [w430]
            tunnel: string[] ["CMin", "F1", "F2", "S1", "S2", "S3", "S4", "S5", "S6", "S7", "S8", "S9", "S10", "S11", "S12", "S13", "S14", "S14F12", "All OFF"] -> [w428] mode=indexing
            tunnel: w264 -> [w429]
            i -> [w425]
            stop <- w442 stop-if-true
            n108 = case shown="0" w425 {
              tunnel: [w468 w471] -> w434
              tunnel: w433 -> [w467 w471]
              tunnel: [w466 w470] -> w432
              tunnel: w431 -> [w465 w470]
              frame 0 {
                w463 = u16 0 items=["Voltage", "Current"] ("Source Mode  (0: Voltage)")
                n109 = call "Configure Output.vi"("Source Mode  (0: Voltage)"=w463, "error in (no error)"=w467, "Output Level (0)"=0.0, "VISA resource name"=w465) -> ("error out"=w469:errorcluster, "VISA resource name out"=w461:refnum<visa-resource-name>)  [unwired: 6 in]
                n110 = call "Enable Output.vi"("error in (no error)"=w469, "Enable Output (T: Enable)"=TRUE, "VISA resource name"=w461) -> ("error out"=w468:errorcluster, "VISA resource name out"=w466:refnum<visa-resource-name>)  [unwired: 7 in]
              }
              frame 1, Default {
              }
            }
            n111 = call "WSVCAP SHL Host TL RFFE Write - Multiple DUTs - Common Data.vi"("Data Out"=w435, "error in"=w434) -> ("error out"=w436:errorcluster)  [unwired: 13 in]
            n112 = case shown="1..3" w425 {
              tunnel: [1 w460] -> w456
              tunnel: w446 -> [_ w459]
              frame 0, Default {
              }
              frame 1..3 {
                n113 = Array Size(array=w459) -> (size(s)=w460:i32)
              }
            }
            n114 = call "Delay T4.vi"("milliseconds to wait"=u32 100, "error in (no error)"=w436) -> ("error out"=w448:errorcluster)  [unwired: 9 in]
            n115 = for {
              N: w456 -> [_]
              tunnel: w446 -> [w530]
              tunnel: w438 -> [w519]
              tunnel: [w528] -> w427
              tunnel: w448 -> [w527]
              tunnel: [w523] -> w457
              tunnel: w455 -> [w505]
              tunnel: w454 -> [w512]
              tunnel: w453 -> [w511]
              tunnel: w452 -> [w510]
              tunnel: w451 -> [w509]
              tunnel: w428 -> [w508]
              tunnel: [w503] -> w449
              tunnel: w432 -> [w495]
              tunnel: w445 -> [w494]
              tunnel: [w491] -> w443
              tunnel: w441 -> [w489]
              tunnel: w437 -> [w488]
              tunnel: w430 -> [w487]
              tunnel: w429 -> [w486]
              tunnel: w428 -> [w485]
              shift-right: [w476] -> _
              shift-left: dbl[] [] -> [w482]
              tunnel: w425 -> [w473]
              tunnel: w424 -> [w472]
              i -> [w518]
              stop <- w491 stop-if-true
              n116 = flat-sequence {
                tunnel: w530 -> [w593]
                tunnel: w518 -> [w592]
                tunnel: w527 -> [w594]
                tunnel: [w558] -> w524
                tunnel: [w572] -> w522
                tunnel: [w573] -> w521
                tunnel: [w574] -> w520
                tunnel: w518 -> [w578]
                tunnel: [w543] -> w517
                tunnel: [w575] -> w516
                tunnel: [w571] -> w515
                tunnel: [w570] -> w514
                tunnel: [w569] -> w513
                tunnel: w508 -> [w568]
                tunnel: [w568] -> w507
                tunnel: [w567] -> w506
                tunnel: w505 -> [w567]
                tunnel: [w566] -> w504
                tunnel: [w565] -> w501
                tunnel: [w564] -> w500
                tunnel: [w563] -> w499
                tunnel: [w553] -> w498
                tunnel: [w552] -> w497
                tunnel: [w551] -> w496
                tunnel: w495 -> [w550]
                tunnel: w494 -> [w549]
                tunnel: [w549] -> w493
                tunnel: [w548] -> w490
                tunnel: w489 -> [w548]
                tunnel: w473 -> [w546]
                tunnel: w487 -> [w545]
                tunnel: w485 -> [w544]
                tunnel: [w542] -> w484
                tunnel: w482 -> [w541]
                tunnel: [w541] -> w481
                tunnel: w473 -> [w540]
                tunnel: [w540] -> w475
                tunnel: [w692] -> w525
                tunnel: [w694] -> w523
                tunnel: [w693] -> w503
                tunnel: [w691] -> w479
                tunnel: [w690] -> w478
                tunnel: [w689] -> w477
                tunnel: w499 -> [w691]
                tunnel: w500 -> [w690]
                tunnel: w501 -> [w689]
                tunnel: w504 -> [w693]
                tunnel: w506 -> [w676]
                tunnel: w507 -> [w663]
                tunnel: w513 -> [w677]
                tunnel: w514 -> [w678]
                tunnel: w515 -> [w679]
                tunnel: w509 -> [w680]
                tunnel: w516 -> [w681]
                tunnel: w517 -> [w674]
                tunnel: w510 -> [w682]
                tunnel: w511 -> [w683]
                tunnel: w512 -> [w684]
                tunnel: w519 -> [w685]
                tunnel: w520 -> [w686]
                tunnel: w521 -> [w687]
                tunnel: w522 -> [w688]
                tunnel: w524 -> [w694]
                tunnel: w498 -> [w667]
                tunnel: w497 -> [w668]
                tunnel: w496 -> [w666]
                tunnel: w493 -> [w664]
                tunnel: [w664] -> w492
                tunnel: w490 -> [w662]
                tunnel: w488 -> [w661]
                tunnel: w486 -> [w660]
                tunnel: w484 -> [w659]
                tunnel: [w659] -> w483
                tunnel: w481 -> [w658]
                tunnel: [w658] -> w480
                tunnel: w475 -> [w657]
                tunnel: [w657] -> w474
                tunnel: w472 -> [w656]
                frame #0 {
                  w580 = FALSE ("Log (T)")
                  n117 = case shown="1..3" w546 {
                    tunnel: w594 -> [w619 w626]
                    tunnel: w593 -> [w618 _]
                    tunnel: w592 -> [w617 _]
                    tunnel: [w608 w626] -> w576
                    tunnel: [w606 w629] -> w575
                    tunnel: [w605 w624] -> w566
                    tunnel: [w600 0.0] -> w542
                    tunnel: [w604 w625] -> w558
                    tunnel: w550 -> [w602 w625]
                    tunnel: [w598 "0"] -> w543
                    tunnel: [w597 w621] -> w547
                    tunnel: w545 -> [w596 w624]
                    tunnel: w544 -> [w595 w622]
                    frame 1..3 {
                      w611 = u16 0 items=["Voltage", "Current"] ("Source Mode  (0: Voltage)")
                      n118 = Index Array(array=w618, index=w617) -> (element=w600:dbl)
                      n119 = call "Configure Output.vi"("Source Mode  (0: Voltage)"=w611, "error in (no error)"=w619, "Compliance  Level (0.1)"="VSA_IDD(A)", "Output Level (0)"=w600, "VISA resource name"=w602) -> ("error out"=w615:errorcluster, "VISA resource name out"=w613:refnum<visa-resource-name>)  [unwired: 5 in]
                      n120 = call "Enable Output.vi"("error in (no error)"=w615, "Enable Output (T: Enable)"=TRUE, "VISA resource name"=w613) -> ("error out"=w616:errorcluster, "VISA resource name out"=w604:refnum<visa-resource-name>)  [unwired: 7 in]
                      n121 = Number To Fractional String(number=w600, precision (6)=i16 2) -> (F-format string=w598:string)  [unwired: 2 in]
                      n122 = call "Delay T4.vi"("milliseconds to wait"=u32 50, "error in (no error)"=w616) -> ("error out"=w603:errorcluster)  [unwired: 9 in]
                      n123 = Concatenate Strings(w595, "_VSA Sweeping Voltage... ", w598) -> (w597:string)
                      n124 = call "Ke2000 Reading MilAmp.vi"("error in (no error)"=w603, "VISA resource name"=w596) -> ("error out"=w608:errorcluster, "uA"=w607:string, "VISA resource name out"=w605:refnum<visa-resource-name>)  [unwired: 7 in]
                      n125 = for {
                        N: 16 -> [_]
                        tunnel: w607 -> [w620]
                        tunnel: [w620] -> w606 mode=indexing
                      }
                    }
                    frame 0, Default {
                      n126 = Concatenate Strings(w622, "_No VSA Sweeping Voltage... ") -> (w621:string)
                      n127 = for {
                        N: 16 -> [_]
                        tunnel: "0" ("uA") -> [w632]
                        tunnel: [w632] -> w629 mode=indexing
                      }
                    }
                  }
                  "CP Current(uA)" <- w575
                  n128 = local write "STATUS"(w547) -> ()
                  n129 = call "WS1050 16 DUT AD7747 READ.vi"("error in"=w576, "Log (T)"=w580, "DUT Mask Mode (All)"=WSVCAP_SHL_I2C_DUT_Mask_Mode_Enum."C1") -> ("error out"=w589:errorcluster, "AD7747 Values"=w591:string[][])  [unwired: 7 in]
                  n130 = for {
                    tunnel: w591 -> [w654] mode=indexing
                    tunnel: [w652] -> w559 mode=indexing
                    tunnel: w589 -> [w653]
                    tunnel: [w653] -> w588
                    n131 = Index Array(array=w654, index=1) -> (element=w652:string)
                  }
                  n132 = call "WS1050 16 DUT AD7747 READ.vi"("error in"=w588, "Log (T)"=w580, "DUT Mask Mode (All)"=WSVCAP_SHL_I2C_DUT_Mask_Mode_Enum."C2") -> ("error out"=w586:errorcluster, "AD7747 Values"=w585:string[][])  [unwired: 7 in]
                  n133 = for {
                    tunnel: w585 -> [w650] mode=indexing
                    tunnel: [w648] -> w560 mode=indexing
                    tunnel: w586 -> [w649]
                    tunnel: [w649] -> w584
                    n134 = Index Array(array=w650, index=3) -> (element=w648:string)
                  }
                  n135 = call "WS1050 16 DUT AD7747 READ.vi"("error in"=w584, "Log (T)"=w580, "DUT Mask Mode (All)"=WSVCAP_SHL_I2C_DUT_Mask_Mode_Enum."C3") -> ("error out"=w582:errorcluster, "AD7747 Values"=w581:string[][])  [unwired: 7 in]
                  n136 = for {
                    tunnel: w581 -> [w646] mode=indexing
                    tunnel: [w644] -> w577 mode=indexing
                    tunnel: w582 -> [w645]
                    tunnel: [w645] -> w579
                    n137 = Index Array(array=w646, index=5) -> (element=w644:string)
                  }
                  n138 = case shown="0" w578 {
                    tunnel: w579 -> [w636 w643]
                    tunnel: [w636 w643] -> w554
                    tunnel: w577 -> [w633 w640]
                    tunnel: w560 -> [w634 w641]
                    tunnel: w559 -> [w635 w642]
                    tunnel: [w635 w642] -> w572
                    tunnel: [w634 w641] -> w573
                    tunnel: [w633 w640] -> w574
                    tunnel: [w633 w639] -> w557
                    tunnel: [w634 w638] -> w556
                    tunnel: [w635 w637] -> w555
                    frame 0 {
                      "VSA_C3_T0" <- w633
                      "VSA_C2_T0" <- w634
                      "VSA_C1_T0" <- w635
                    }
                    frame 1, Default {
                      n139 = local read "VSA_C1_T0"() -> (w637:string[])
                      n140 = local read "VSA_C2_T0"() -> (w638:string[])
                      n141 = local read "VSA_C3_T0"() -> (w639:string[])
                    }
                  }
                  n142 = Build Array(w559, w560, w577) -> (w561:string[][])
                  n143 = Transpose 2D Array(2D array=w561) -> (transposed array=→"VSA_Value(pF)":string[][])
                  n144 = call "WS1050 VSA_Delta C Calculation.vi"("error in (no error)"=w554, "VSA_T"=w572, "VSA_T0"=w555) -> ("error out"=w553:errorcluster, 2:"VSA Delta C(pF)"=w563:dbl[], 3:"VSA Delta C(pF)"=w571:string[])  [unwired: 6 in]
                  n145 = call "WS1050 VSA_Delta C Calculation.vi"("error in (no error)"=w554, "VSA_T"=w573, "VSA_T0"=w556) -> ("error out"=w552:errorcluster, 2:"VSA Delta C(pF)"=w564:dbl[], 3:"VSA Delta C(pF)"=w570:string[])  [unwired: 6 in]
                  n146 = call "WS1050 VSA_Delta C Calculation.vi"("error in (no error)"=w554, "VSA_T"=w574, "VSA_T0"=w557) -> ("error out"=w551:errorcluster, 2:"VSA Delta C(pF)"=w565:dbl[], 3:"VSA Delta C(pF)"=w569:string[])  [unwired: 6 in]
                }
                frame #1 {
                  n147 = Get Date/Time In Seconds() -> (seconds since 1Jan1904=w673:timestamp)
                  n148 = Concatenate Strings(w663, w676) -> (w675:string)
                  n149 = Get Date/Time String(seconds (now)=w673, want seconds? (F)=TRUE) -> (date string=→"date string":string, time string=→"Previous Time":string)  [unwired: 1 in]
                  n150 = Merge Errors(w667, w668, w666) -> (w665:errorcluster)
                  n151 = call "WS1050_16 DUT VSA Save Data Ver1.0.vi"("TMN DC\\CAP Data Log File Path"=w685, "Lot#"=w684, "VSA_Delta C1(pF)"=w679, "Wafer#"=w683, "File Name"=w680, "VSA_Delta C2(pF)"=w678, "error in"=w665, "Comment"=w675, "CP Current(uA)"=w681, "VSA_IDD(A)"="NA", "HD Time(Min)"=w656, "Driver"=w663, "VSA_C1"=w688, "CP HD (V)"=w662, "VSA_C2"=w687, "SN"=w682, "VSA_C3"=w686, "Test Program"=w661, "Voltage(V)"=w674, "Stress Voltage(V)"=w660, "VSA_Delta C3(pF)"=w677) -> ("error out"=w692:errorcluster)  [unwired: 6 in]
                }
              }
              n152 = Increment(x=w518) -> (x+1=→"Running Loops":i32)
              n153 = Build Array (concatenate)(w480, w483) -> (w476:dbl[])
              n154 = case shown="1..3" w474 {
                tunnel: w479 -> [w539 _]
                tunnel: w478 -> [w536 _]
                tunnel: w476 -> [w534 _]
                tunnel: w477 -> [w533 _]
                tunnel: w476 -> [w532 _]
                tunnel: w476 -> [w531 _]
                frame 1..3 {
                  n155 = Bundle(w531, "VSA Delta C(pF)"=w536) -> (→"Plot VSA Delta C2":cluster{dbl[], "VSA Delta C(pF)":dbl[]})  [unwired: 1 in]
                  n156 = Bundle(w534, "VSA Delta C(pF)"=w539) -> (→"Plot VSA Delta C1":cluster{dbl[], "VSA Delta C(pF)":dbl[]})  [unwired: 1 in]
                  n157 = Bundle(w532, "VSA Delta C(pF)"=w533) -> (→"Plot VSA Delta C3":cluster{dbl[], "VSA Delta C(pF)":dbl[]})  [unwired: 1 in]
                }
                frame 0, Default {
                }
              }
              n158 = call "Delay T4.vi"("milliseconds to wait"=u32 10, "error in (no error)"=w525) -> ("error out"=w528:errorcluster)  [unwired: 9 in]
              n159 = Unbundle By Name(w528) -> ("status"=w502:bool)
              n160 = Compound Arithmetic op=OR(w502, w492) -> (w491:bool)
              "VSA Delta C1(pF)" <- w479
              "VSA Delta C2(pF)" <- w478
              "VSA Delta C3(pF)" <- w477
            }
            n161 = Unbundle By Name(w427) -> ("status"=w444:bool)
            n162 = call "Delay T4.vi"("milliseconds to wait"=u32 10, "error in (no error)"=w427) -> ("error out"=w440:errorcluster)  [unwired: 9 in]
            n163 = Or(x=w444, y=w443) -> (x .or. y?=w442:bool)
          }
          n164 = flat-sequence {
            tunnel: w291 -> [w320]
            tunnel: [w320] -> w290
            tunnel: w288 -> [w318]
            tunnel: [w319] -> w289
            frame #0 {
              n165 = Greater Or Equal?(x=w318, y="Set HD Time \nto Complete(Min)") -> (x >= y?=w319:bool)
              "HD Time\nCompleted(Min)" <- w318
            }
          }
          n166 = Unbundle By Name(w290) -> ("status"=w293:bool)
          n167 = call "Delay T4.vi"("milliseconds to wait"=u32 50, "error in (no error)"=w290) -> ("error out"=w306:errorcluster)  [unwired: 9 in]
          n168 = Compound Arithmetic op=OR(w289, w293, w283) -> (w260:bool)
        }
        n169 = VISA Write(VISA resource name=w241, write buffer="SOUR:FUNC VOLT;VOLT:MODE FIX;RANG 100;LEV 0.0;:SENS:FUNC \"CURR\";CURR:PROT 60E-3;RANG 100E-3;:OUTP ON", error in (no error)=w232) -> (VISA resource name out=w245:refnum<visa-resource-name>, error out=w236:errorcluster)  [unwired: 1 out]
        n170 = for {
          tunnel: w235 -> [w258]
          tunnel: w237 -> [w255] mode=indexing
          shift-right: [w253] -> w231
          shift-left: w236 -> [w259]
          tunnel: [w251] -> w234
          n171 = call "E3631A_Voltage Controller.vi"("VISA resource name"=w258, "Channel Controller"=w255, "Voltage 1"=0.0, "Voltage 2"=3.3, "error in (no error)"=w259, "Voltage 3"=-3.3) -> ("VISA resource name out"=w251:refnum<visa-resource-name>, "error out"=w254:errorcluster)  [unwired: 8 in]
          n172 = call "Delay T4.vi"("milliseconds to wait"=u32 100, "error in (no error)"=w254) -> ("error out"=w253:errorcluster)  [unwired: 9 in]
        }
        n173 = flat-sequence {
          tunnel: w231 -> [w695]
          tunnel: [w695] -> w230
          frame #0 {
            n174 = local write "STATUS"("Idle...." ("STATUS")) -> ()
            n175 = One Button Dialog(message="Test Completed") -> ()  [unwired: 1 in, 1 out]
          }
        }
      }
      frame True {
        w698 = FALSE
      }
    }
    n176 = Wait Until Next ms Multiple(millisecond multiple=u32 100) -> ()  [unwired: 1 out]
    n177 = local write "Abort"(w54) -> ()
    n178 = local write "stop"(w55) -> ()
    n179 = Unbundle By Name(w57) -> ("status"=w73:bool)
    n180 = Compound Arithmetic op=OR(w50, w73, w65) -> (w72:bool)
  }
  "Ke2000 Out" <- w23
  "PS1 Out" <- w22
  n181 = local write "Abort"(w7) -> ()
  n182 = local write "stop"(w7) -> ()
  n183 = case shown="True" w20 {
    tunnel: [w703 w705] -> w6
    tunnel: w14 -> [w703 w704]
    frame False {
    }
    frame True {
      n184 = flat-sequence {
        tunnel: w704 -> [w708]
        tunnel: [w707] -> w705
        frame #0 {
          n185 = local write "Online"(FALSE ("Online")) -> ()
          n186 = call "WSVCAP SHL Host TL Close.vi"("error in"=w708) -> ("error out"=w707:errorcluster)  [unwired: 14 in]
        }
      }
    }
  }
  "error out" <- w6
  n187 = VISA Write(VISA resource name=w15, write buffer="SOUR:FUNC VOLT;VOLT:MODE FIX;RANG 100;LEV 0.0;:SENS:FUNC \"CURR\";CURR:PROT 60E-3;RANG 100E-3;:OUTP OFF", error in (no error)=w14) -> (VISA resource name out=→"VISA resource name out":refnum<visa-resource-name>, error out=→"error out 2":errorcluster)  [unwired: 1 out]
